vi "日期时间字符串转换秒数加一.vi"(11 "data[0]":string) -> (3 "日期/时间字符串":string)   [LabVIEW 2016, in "数据传输系统-02.lvlib"]
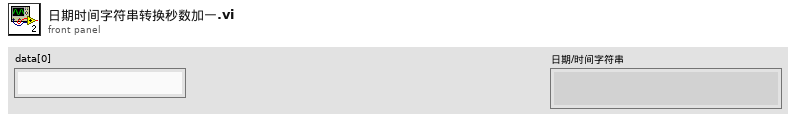
[diagram p1: front panel]
types:
  T1 = typedef "LVDateTimeRec.ctl" = cluster{"秒数的小数部分":dbl, "秒":i32, "分":i32, "时":i32, "日":i32, "月":i32, "年":i32, "天数（周）":i32, "天数（年）":i32, "DST":i32}
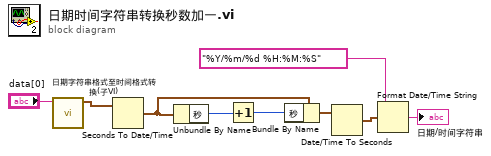
[diagram p0: block diagram]
diagram:
  n1 = call "日期字符串格式至时间格式转换(子VI).vi"("data[0]"="data[0]") -> ("time stamp"=w3:timestamp)  [unwired: 10 in]
  n2 = Seconds To Date/Time(time stamp (now)=w3) -> (date time rec=w5:T1)  [unwired: 1 in]
  n3 = Unbundle By Name(w5) -> ("秒"=w4:i32)
  n4 = Increment(x=w4) -> (x+1=w6:i32)
  n5 = Bundle By Name(cluster=w5, "秒"=w6) -> (w8:T1)
  n6 = Date/Time To Seconds(2:w8) -> (0:w7:timestamp)  [unwired: 1 in]
  n7 = Format Date/Time String(time format string (%c)="%Y/%m/%d %H:%M:%S" ("时间格式字符串(%c)"), seconds (now)=w7) -> (date/time string=→"日期/时间字符串":string)  [unwired: 1 in]
